vi "Do.vi"(8 "error in":errorcluster, 10 "Actor in":refnum<class "Actor.lvclass">, 11 "DS Reply Msg in":refnum<class "Reply Msg DataSocket.lvclass">) -> (0 "error out":errorcluster, 2 "Actor out":refnum<class "Actor.lvclass">)   [LabVIEW 2023, in "Reply Msg DataSocket.lvclass"]
uses:
  Reply Msg DataSocket.lvclass
  <vilib>/ActorFramework/Actor/Actor.lvclass
  HAL/HAL GOOP4/Reply Protocol Manager/Reply Protocol Manager.lvclass
  Reply Msg DataSocket.lvclass/Reply Msg DataSocket.ctl
  HAL/HAL GOOP4/Reply Protocol/Reply Protocol DataSocket/Reply Protocol DataSocket.lvclass
  <vilib>/ErrorRing/Error Ring.xnode
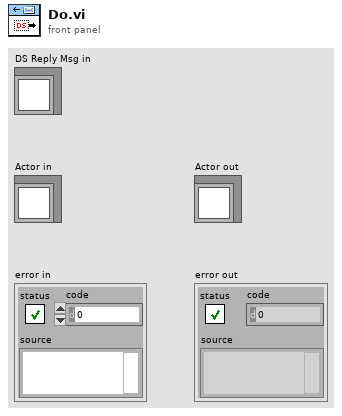
[diagram p1: front panel]
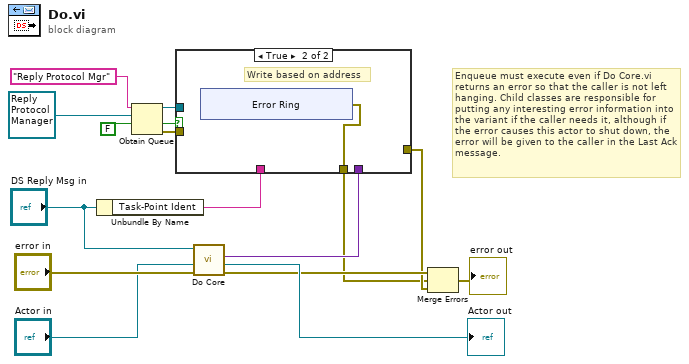
[diagram p0: block diagram]
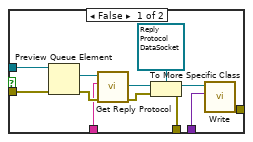
[diagram p2: hidden frame]
diagram:
  # "Enqueue must execute even if Do Core.vi returns an error so that the caller is not left hanging. Child classes are responsible for putting any interesting error information into the variant if the caller needs it, although if the error causes this actor to shut down, the error will be given to the caller in the Last Ack message."
  n1 = Unbundle By Name("DS Reply Msg in") -> ("Task-Point Ident"=w5:string)
  n2 = Obtain Queue(name (unnamed)="Reply Protocol Mgr", element data type=refnum<class "Reply Protocol Manager.lvclass"> refnum ("HAL GOOP4.lvlib:Reply Protocol Manager"), create if not found? (T)=FALSE) -> (queue out=w10:refnum<queue>, created new?=w1:bool, error out=w9:errorcluster)  [unwired: 2 in]
  n3 = call-dynamic "Do Core.vi"("error in"="error in", "Actor in"="Actor in", "DS Reply Msg in"="DS Reply Msg in") -> ("error out"=w12:errorcluster, "Actor out"=→"Actor out":refnum<class "Actor.lvclass">, "Reply"=w4:variant)  [unwired: 6 in]
  n4 = case shown="True" w1 {
    tunnel: w10 -> [w28 _]
    tunnel: w9 -> [w27 _]
    tunnel: w5 -> [w24 _]
    tunnel: w4 -> [w23 _]
    tunnel: [w18 _] -> w3
    tunnel: [w17 w29] -> w2
    frame False {
      n5 = Preview Queue Element(queue=w28, error in (no error)=w27) -> (element=w25:refnum<class "Reply Protocol Manager.lvclass">, error out=w26:errorcluster)  [unwired: 1 in, 2 out]
      n6 = call "Get Reply Protocol.vi"("Error In"=w26, "Identifier"=w24, "reference in"=w25) -> ("Error Out"=w20:errorcluster, "Reply Protocol Base"=w22:refnum<class "Reply Protocol Base.lvclass">)  [unwired: 6 in, 1 out]
      n7 = To More Specific Class(target class=refnum<class "Reply Protocol DataSocket.lvclass"> refnum ("HAL GOOP4.lvlib:Reply Protocol DataSocket.lvclass"), reference=w22, error in=w20) -> (specific class reference=w21:refnum<class "Reply Protocol DataSocket.lvclass">, error out=w17:errorcluster)
      n8 = call-dynamic "Write.vi"("Variant"=w23, "Reply Protocol DataSocket in"=w21) -> ("error out"=w18:errorcluster)  [unwired: 7 in, 2 out]
    }
    frame True {
      # "Write based on address"
      n9 = xnode "Error Ring"() -> ("error out"=w29:errorcluster)
    }
  }
  n10 = Merge Errors(w12, w2, w3) -> (→"error out":errorcluster)
